vi "Random Data one Line.vi"() -> ()   [LabVIEW 2025]
uses:
  <vilib>/numeric/Random Number (Range) DBL.vi
  <vilib>/Analysis/4window.llb/Gaussian Window (DBL).vi
  <vilib>/Analysis/2dsp.llb/Complex FFT.vi
  <vilib>/Analysis/1siggen.llb/Ramp Pattern by Samples.vi
  <extravilib>/ChannelInstances/Tag-cdb/Instantiate.vi
  <extravilib>/ChannelInstances/Tag-cdb/EndpointRead.vi
  <extravilib>/ChannelInstances/Tag-cdb/Endpoint.vi
  <vilib>/Analysis/NI_AALPro.lvlib
  <vilib>/Analysis/NI_AALBase.lvlib
  <extravilib>/ChannelInstances/Tag-cdb.lvlib
  <vilib>/Analysis/2dsp.llb/Resample (constant to constant, complex single-channel).vi
panel:
  in  "Zoom Range":dbl=100.0 format="%#_13g"
  in  "Wait Time":dbl(slide)=71.49146578212554 scale=1.0..500.0
  in  "Zoom Point Index":i32=13
  in  "Individual Plots \nPer Vector":bool=TRUE
  out "Waveform Graph 2":dbl[][](graph)
  out "XY Graph":cluster{"XY Graph - Light":cdb[]}[](graph)
  out "XY Graph 2":cluster{"XY Graph - Light":cdb[]}[](graph)
  out "Spectrum":dbl[][](graph)
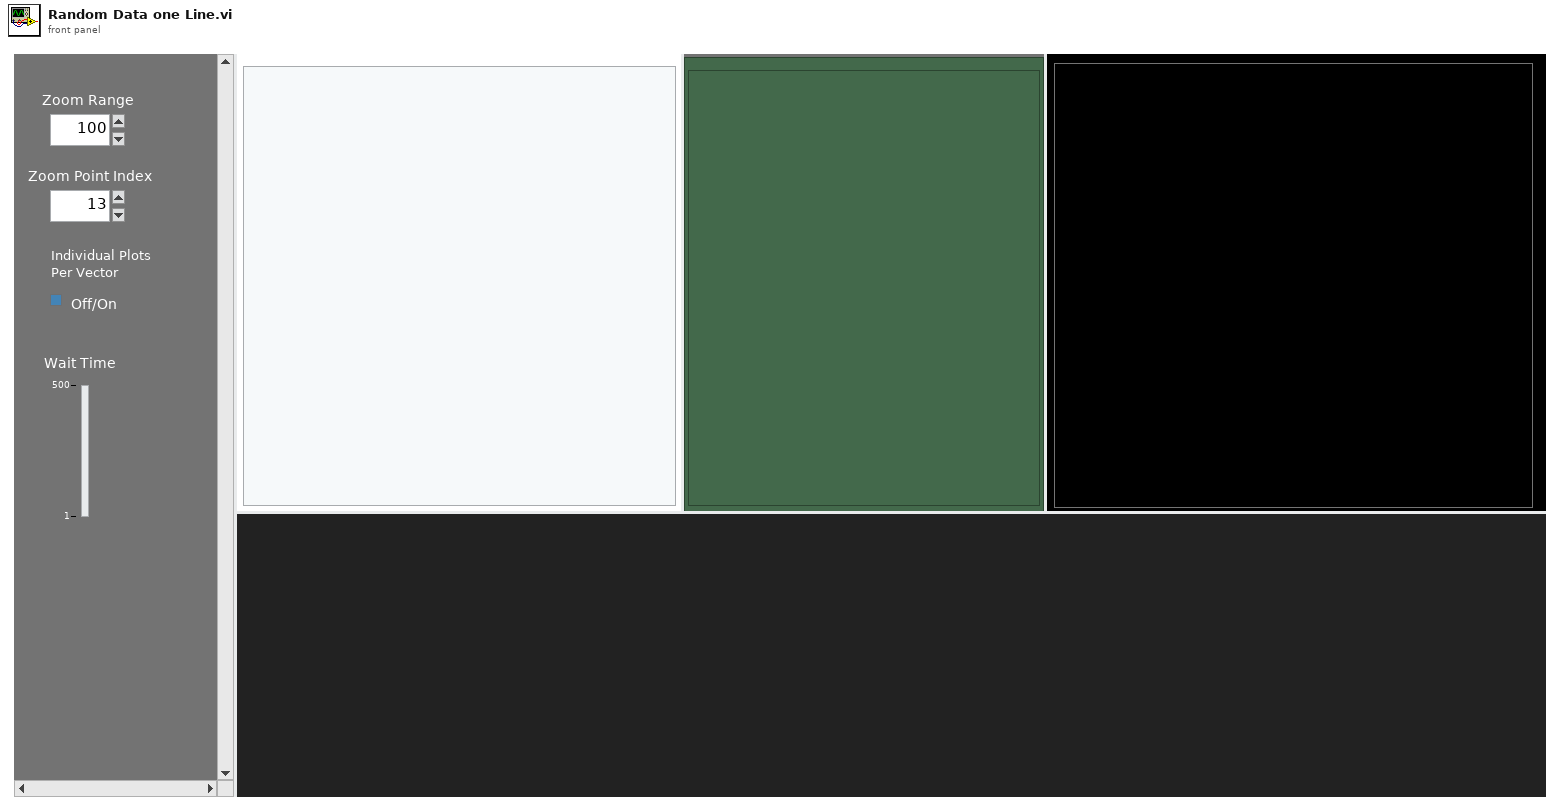
[diagram p1: front panel]
types:
  T1 = typedef "Tag-cdb.lvlib/))Channel.ctl" = refnum<queue>
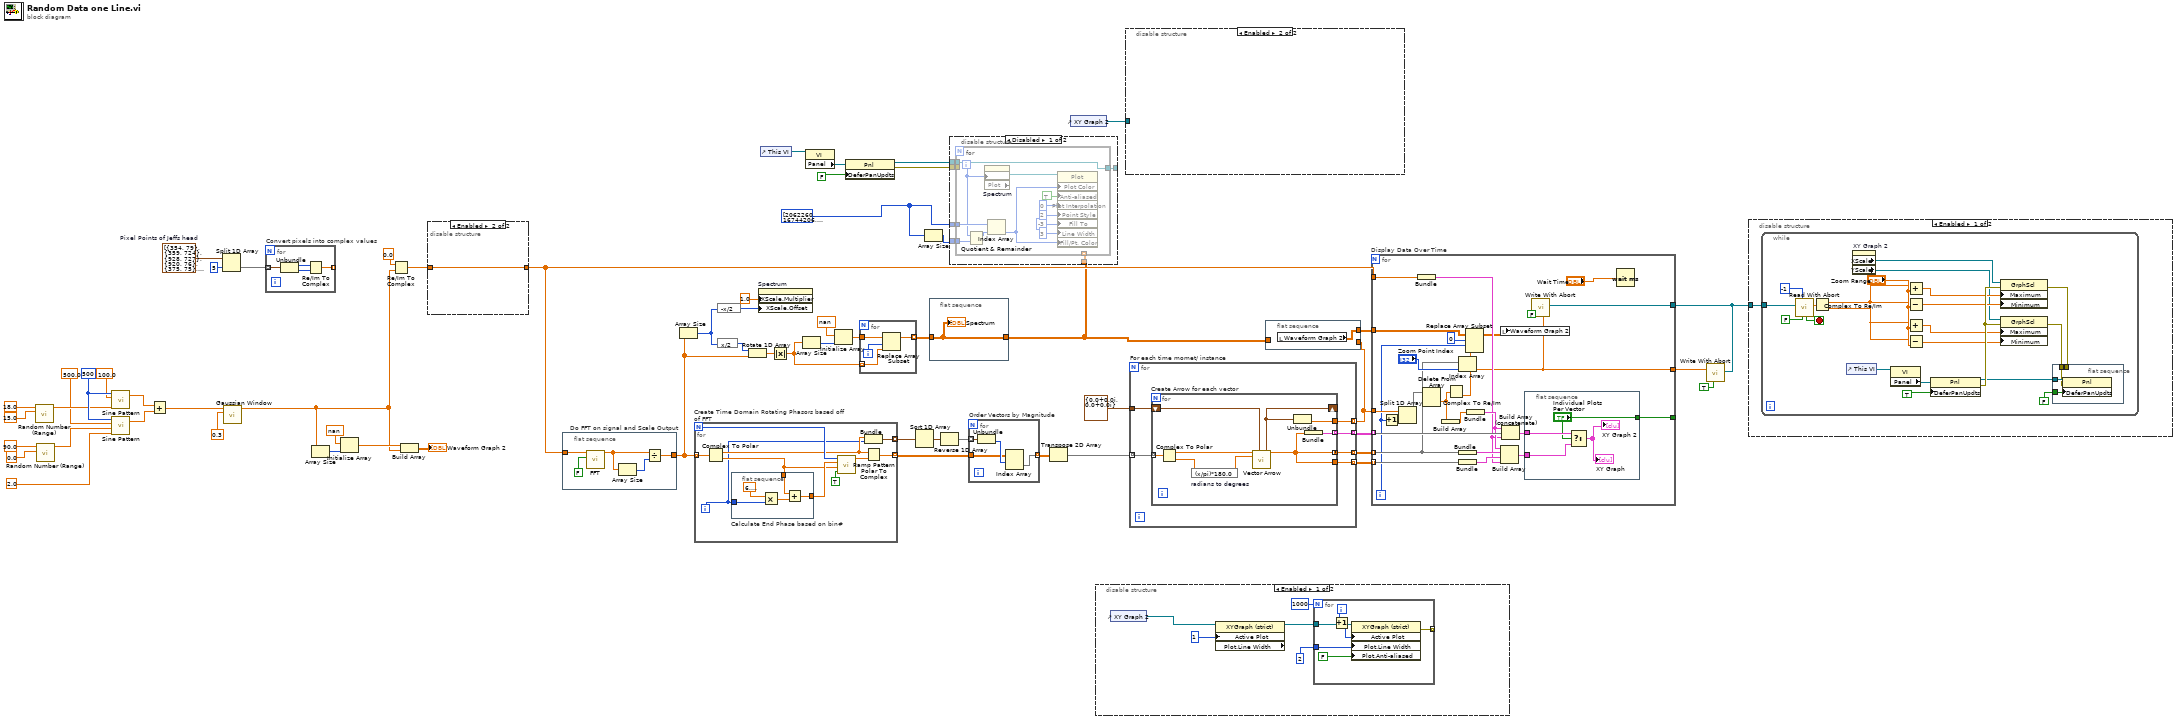
[diagram p0: block diagram]
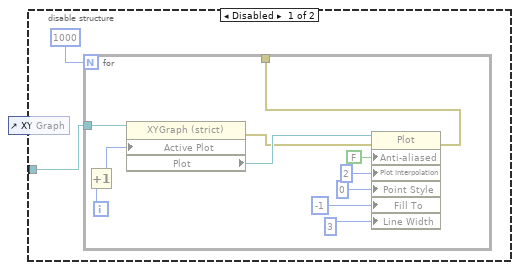
[diagram p3: hidden frame]
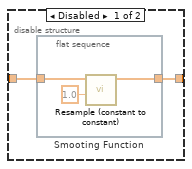
[diagram p5: hidden frame]
diagram:
  w2 = u32[] [2062260, 16744206, 2924588, 14034728, 9725885, 9197131, 14907330, 8355711, 12369186, 1556175] ("Array")
  w43 = 500 ("samples")
  w54 = cluster{"Horizontal":i32, "Vertical":i32}[] [{"Horizontal"=354, "Vertical"=79}, {"Horizontal"=359, "Vertical"=724}, {"Horizontal"=928, "Vertical"=727}, {"Horizontal"=920, "Vertical"=76}, {"Horizontal"=375, "Vertical"=75}, {"Horizontal"=348, "Vertical"=534}, {"Horizontal"=379, "Vertical"=519}, {"Horizontal"=407, "Vertical"=510}, {"Horizontal"=436, "Vertical"=501}, {"Horizontal"=463, "Vertical"=490}, {"Horizontal"=491, "Vertical"=484}, {"Horizontal"=514, "Vertical"=473}, {"Horizontal"=528, "Vertical"=466}, {"Horizontal"=536, "Vertical"=452}, {"Horizontal"=523, "Vertical"=437}, {"Horizontal"=518, "Vertical"=417}, {"Horizontal"=512, "Vertical"=396}, {"Horizontal"=508, "Vertical"=372}, {"Horizontal"=503, "Vertical"=348}, {"Horizontal"=490, "Vertical"=331}, {"Horizontal"=491, "Vertical"=315}, {"Horizontal"=502, "Vertical"=290}, {"Horizontal"=511, "Vertical"=302}, {"Horizontal"=520, "Vertical"=312}, {"Horizontal"=529, "Vertical"=324}, {"Horizontal"=531, "Vertical"=338}, {"Horizontal"=536, "Vertical"=353}, {"Horizontal"=547, "Vertical"=354}, {"Horizontal"=563, "Vertical"=359}, {"Horizontal"=570, "Vertical"=361}, {"Horizontal"=586, "Vertical"=363}, {"Horizontal"=595, "Vertical"=363}, {"Horizontal"=610, "Vertical"=363}, {"Horizontal"=617, "Vertical"=349}, {"Horizontal"=623, "Vertical"=335}, {"Horizontal"=629, "Vertical"=318}, {"Horizontal"=618, "Vertical"=309}, {"Horizontal"=601, "Vertical"=306}, {"Horizontal"=587, "Vertical"=303}, {"Horizontal"=567, "Vertical"=299}, {"Horizontal"=551, "Vertical"=301}, {"Horizontal"=539, "Vertical"=305}, {"Horizontal"=529, "Vertical"=306}, {"Horizontal"=520, "Vertical"=296}, {"Horizontal"=512, "Vertical"=281}, {"Horizontal"=506, "Vertical"=277}, {"Horizontal"=502, "Vertical"=269}, {"Horizontal"=508, "Vertical"=250}, {"Horizontal"=516, "Vertical"=232}, {"Horizontal"=525, "Vertical"=213}, {"Horizontal"=539, "Vertical"=188}, {"Horizontal"=547, "Vertical"=174}, {"Horizontal"=563, "Vertical"=162}, {"Horizontal"=579, "Vertical"=144}, {"Horizontal"=587, "Vertical"=136}, {"Horizontal"=610, "Vertical"=128}, {"Horizontal"=629, "Vertical"=129}, {"Horizontal"=656, "Vertical"=127}, {"Horizontal"=666, "Vertical"=131}, {"Horizontal"=697, "Vertical"=140}, {"Horizontal"=711, "Vertical"=143}, {"Horizontal"=745, "Vertical"=163}, {"Horizontal"=750, "Vertical"=169}, {"Horizontal"=757, "Vertical"=193}, {"Horizontal"=771, "Vertical"=200}, {"Horizontal"=767, "Vertical"=224}, {"Horizontal"=774, "Vertical"=238}, {"Horizontal"=779, "Vertical"=268}, {"Horizontal"=783, "Vertical"=284}, {"Horizontal"=765, "Vertical"=286}, {"Horizontal"=746, "Vertical"=291}, {"Horizontal"=737, "Vertical"=300}, {"Horizontal"=718, "Vertical"=302}, {"Horizontal"=696, "Vertical"=299}, {"Horizontal"=679, "Vertical"=302}, {"Horizontal"=655, "Vertical"=304}, {"Horizontal"=650, "Vertical"=306}, {"Horizontal"=636, "Vertical"=308}, {"Horizontal"=620, "Vertical"=309}, {"Horizontal"=643, "Vertical"=317}, {"Horizontal"=651, "Vertical"=334}, {"Horizontal"=656, "Vertical"=342}, {"Horizontal"=664, "Vertical"=358}, {"Horizontal"=674, "Vertical"=367}, {"Horizontal"=689, "Vertical"=360}, {"Horizontal"=712, "Vertical"=361}, {"Horizontal"=731, "Vertical"=353}, {"Horizontal"=738, "Vertical"=346}, {"Horizontal"=747, "Vertical"=326}, {"Horizontal"=744, "Vertical"=315}, {"Horizontal"=751, "Vertical"=304}, {"Horizontal"=759, "Vertical"=294}, {"Horizontal"=773, "Vertical"=291}, {"Horizontal"=785, "Vertical"=286}, {"Horizontal"=770, "Vertical"=296}, {"Horizontal"=778, "Vertical"=306}, {"Horizontal"=776, "Vertical"=317}, {"Horizontal"=775, "Vertical"=326}, {"Horizontal"=773, "Vertical"=340}, {"Horizontal"=771, "Vertical"=353}, {"Horizontal"=765, "Vertical"=360}, {"Horizontal"=762, "Vertical"=383}, {"Horizontal"=763, "Vertical"=406}, {"Horizontal"=761, "Vertical"=420}, {"Horizontal"=778, "Vertical"=434}, {"Horizontal"=782, "Vertical"=446}, {"Horizontal"=798, "Vertical"=459}, {"Horizontal"=811, "Vertical"=468}, {"Horizontal"=829, "Vertical"=476}, {"Horizontal"=847, "Vertical"=485}, {"Horizontal"=865, "Vertical"=489}, {"Horizontal"=878, "Vertical"=495}, {"Horizontal"=891, "Vertical"=500}, {"Horizontal"=903, "Vertical"=505}, {"Horizontal"=926, "Vertical"=511}, {"Horizontal"=912, "Vertical"=713}, {"Horizontal"=794, "Vertical"=706}, {"Horizontal"=812, "Vertical"=684}, {"Horizontal"=820, "Vertical"=665}, {"Horizontal"=829, "Vertical"=650}, {"Horizontal"=835, "Vertical"=631}, {"Horizontal"=844, "Vertical"=612}, {"Horizontal"=853, "Vertical"=594}, {"Horizontal"=859, "Vertical"=579}, {"Horizontal"=851, "Vertical"=571}, {"Horizontal"=840, "Vertical"=563}, {"Horizontal"=827, "Vertical"=556}, {"Horizontal"=837, "Vertical"=547}, {"Horizontal"=849, "Vertical"=536}, {"Horizontal"=851, "Vertical"=528}, {"Horizontal"=844, "Vertical"=519}, {"Horizontal"=840, "Vertical"=498}, {"Horizontal"=832, "Vertical"=485}, {"Horizontal"=829, "Vertical"=473}, {"Horizontal"=758, "Vertical"=419}, {"Horizontal"=760, "Vertical"=437}, {"Horizontal"=762, "Vertical"=465}, {"Horizontal"=755, "Vertical"=482}, {"Horizontal"=751, "Vertical"=506}, {"Horizontal"=744, "Vertical"=525}, {"Horizontal"=739, "Vertical"=547}, {"Horizontal"=731, "Vertical"=561}, {"Horizontal"=726, "Vertical"=580}, {"Horizontal"=723, "Vertical"=604}, {"Horizontal"=719, "Vertical"=620}, {"Horizontal"=715, "Vertical"=637}, {"Horizontal"=706, "Vertical"=665}, {"Horizontal"=705, "Vertical"=683}, {"Horizontal"=701, "Vertical"=700}, {"Horizontal"=698, "Vertical"=709}, {"Horizontal"=694, "Vertical"=718}, {"Horizontal"=689, "Vertical"=722}, {"Horizontal"=676, "Vertical"=712}, {"Horizontal"=674, "Vertical"=695}, {"Horizontal"=667, "Vertical"=682}, {"Horizontal"=671, "Vertical"=666}, {"Horizontal"=660, "Vertical"=646}, {"Horizontal"=664, "Vertical"=635}, {"Horizontal"=668, "Vertical"=624}, {"Horizontal"=675, "Vertical"=620}, {"Horizontal"=679, "Vertical"=623}, {"Horizontal"=692, "Vertical"=630}, {"Horizontal"=693, "Vertical"=633}, {"Horizontal"=698, "Vertical"=635}, {"Horizontal"=711, "Vertical"=628}, {"Horizontal"=721, "Vertical"=615}, {"Horizontal"=726, "Vertical"=586}, {"Horizontal"=746, "Vertical"=531}, {"Horizontal"=758, "Vertical"=482}, {"Horizontal"=753, "Vertical"=456}, {"Horizontal"=740, "Vertical"=475}, {"Horizontal"=727, "Vertical"=490}, {"Horizontal"=713, "Vertical"=503}, {"Horizontal"=696, "Vertical"=531}, {"Horizontal"=683, "Vertical"=529}, {"Horizontal"=671, "Vertical"=538}, {"Horizontal"=659, "Vertical"=550}, {"Horizontal"=642, "Vertical"=552}, {"Horizontal"=628, "Vertical"=553}, {"Horizontal"=602, "Vertical"=550}, {"Horizontal"=592, "Vertical"=529}, {"Horizontal"=586, "Vertical"=528}, {"Horizontal"=579, "Vertical"=519}, {"Horizontal"=570, "Vertical"=508}, {"Horizontal"=564, "Vertical"=492}, {"Horizontal"=557, "Vertical"=481}, {"Horizontal"=553, "Vertical"=470}, {"Horizontal"=548, "Vertical"=456}, {"Horizontal"=540, "Vertical"=468}, {"Horizontal"=541, "Vertical"=485}, {"Horizontal"=542, "Vertical"=508}, {"Horizontal"=539, "Vertical"=527}, {"Horizontal"=544, "Vertical"=555}, {"Horizontal"=543, "Vertical"=588}, {"Horizontal"=539, "Vertical"=614}, {"Horizontal"=539, "Vertical"=631}, {"Horizontal"=539, "Vertical"=656}, {"Horizontal"=542, "Vertical"=673}, {"Horizontal"=539, "Vertical"=687}, {"Horizontal"=545, "Vertical"=712}, {"Horizontal"=542, "Vertical"=723}, {"Horizontal"=547, "Vertical"=727}, {"Horizontal"=572, "Vertical"=724}, {"Horizontal"=578, "Vertical"=696}, {"Horizontal"=578, "Vertical"=682}, {"Horizontal"=586, "Vertical"=659}, {"Horizontal"=588, "Vertical"=638}, {"Horizontal"=593, "Vertical"=613}, {"Horizontal"=601, "Vertical"=601}, {"Horizontal"=609, "Vertical"=614}, {"Horizontal"=613, "Vertical"=626}, {"Horizontal"=625, "Vertical"=640}, {"Horizontal"=614, "Vertical"=670}, {"Horizontal"=610, "Vertical"=680}, {"Horizontal"=604, "Vertical"=701}, {"Horizontal"=604, "Vertical"=706}, {"Horizontal"=602, "Vertical"=710}, {"Horizontal"=597, "Vertical"=718}, {"Horizontal"=596, "Vertical"=718}, {"Horizontal"=597, "Vertical"=718}, {"Horizontal"=596, "Vertical"=717}, {"Horizontal"=596, "Vertical"=717}, {"Horizontal"=597, "Vertical"=715}, {"Horizontal"=598, "Vertical"=709}, {"Horizontal"=598, "Vertical"=709}, {"Horizontal"=597, "Vertical"=709}, {"Horizontal"=573, "Vertical"=709}, {"Horizontal"=585, "Vertical"=684}, {"Horizontal"=591, "Vertical"=655}, {"Horizontal"=597, "Vertical"=623}, {"Horizontal"=599, "Vertical"=596}, {"Horizontal"=588, "Vertical"=609}, {"Horizontal"=577, "Vertical"=631}, {"Horizontal"=566, "Vertical"=639}, {"Horizontal"=539, "Vertical"=591}, {"Horizontal"=545, "Vertical"=484}, {"Horizontal"=563, "Vertical"=510}, {"Horizontal"=582, "Vertical"=478}, {"Horizontal"=595, "Vertical"=486}, {"Horizontal"=606, "Vertical"=492}, {"Horizontal"=641, "Vertical"=500}, {"Horizontal"=652, "Vertical"=495}, {"Horizontal"=660, "Vertical"=496}, {"Horizontal"=684, "Vertical"=488}, {"Horizontal"=695, "Vertical"=478}, {"Horizontal"=701, "Vertical"=471}, {"Horizontal"=695, "Vertical"=427}, {"Horizontal"=683, "Vertical"=432}, {"Horizontal"=660, "Vertical"=437}, {"Horizontal"=651, "Vertical"=441}, {"Horizontal"=635, "Vertical"=438}, {"Horizontal"=615, "Vertical"=436}, {"Horizontal"=605, "Vertical"=434}, {"Horizontal"=594, "Vertical"=429}, {"Horizontal"=587, "Vertical"=422}, {"Horizontal"=591, "Vertical"=415}, {"Horizontal"=603, "Vertical"=422}, {"Horizontal"=619, "Vertical"=424}, {"Horizontal"=629, "Vertical"=424}, {"Horizontal"=645, "Vertical"=423}, {"Horizontal"=653, "Vertical"=422}, {"Horizontal"=661, "Vertical"=422}, {"Horizontal"=679, "Vertical"=421}, {"Horizontal"=686, "Vertical"=419}, {"Horizontal"=687, "Vertical"=418}, {"Horizontal"=705, "Vertical"=409}, {"Horizontal"=696, "Vertical"=390}, {"Horizontal"=687, "Vertical"=382}, {"Horizontal"=676, "Vertical"=378}, {"Horizontal"=664, "Vertical"=386}, {"Horizontal"=648, "Vertical"=397}, {"Horizontal"=642, "Vertical"=397}, {"Horizontal"=626, "Vertical"=394}, {"Horizontal"=616, "Vertical"=389}, {"Horizontal"=605, "Vertical"=383}, {"Horizontal"=606, "Vertical"=375}, {"Horizontal"=616, "Vertical"=361}, {"Horizontal"=624, "Vertical"=344}, {"Horizontal"=631, "Vertical"=329}, {"Horizontal"=641, "Vertical"=322}, {"Horizontal"=648, "Vertical"=330}, {"Horizontal"=657, "Vertical"=349}, {"Horizontal"=669, "Vertical"=360}, {"Horizontal"=681, "Vertical"=369}]  # Pixel Points of Jeffs head
  n1 = call-poly <vilib>:"Random Number (Range).vi"("lower bound (0)"=15.0, "upper bound (100)"=18.0) -> ("number"=w38:dbl)  [unwired: 9 in]
  n2 = call-poly <vilib>:"Random Number (Range).vi"("lower bound (0)"=0.0, "upper bound (100)"=90.0) -> ("number"=w22:dbl)  [unwired: 9 in]
  n3 = call <vilib>:"Sine Pattern.vi"("cycles"=w38, "amplitude"=100.0, "samples"=w43) -> ("Sinusoidal Pattern"=w41:dbl[])  [unwired: 1 in, 1 out]
  n4 = call <vilib>:"Sine Pattern.vi"("cycles"=2.0, "phase(degrees)"=w22, "amplitude"=500.0, "samples"=w43) -> ("Sinusoidal Pattern"=w40:dbl[])  [unwired: 1 out]
  n5 = Add(x=w41, y=w40) -> (x+y=w26:dbl[])
  n6 = Split 1D Array(array=w54, index=5) -> (second subarray=w53:cluster{"Horizontal":i32, "Vertical":i32}[])  [unwired: 1 out]
  n7 = call-poly <vilib>:"Gaussian Window.vi"("standard deviation"=0.3, "X"=w26) -> ("Windowed X"=w17:dbl[])  [unwired: 8 in, 1 out]
  n8 = for "Convert pixels into complex values" {
    tunnel: w53 -> [w64] mode=indexing
    tunnel: [w61] -> _ mode=indexing
    n9 = Unbundle(w64) -> ("Horizontal"=w63:i32, "Vertical"=w62:i32)
    n10 = Re/Im To Complex(1:w62, 2:w63) -> (0:w61:cdb)
  }
  n11 = Array Size(array=w17) -> (size(s)=w18:i32)
  n12 = Initialize Array(nan ("element"), w18) -> (w19:dbl[])
  n13 = Re/Im To Complex(1:w17, 2:0.0 ("cycles")) -> (0:w16:cdb[])
  n14 = Build Array(w19, w17) -> (→"Waveform Graph 2":dbl[][])
  n15 = disable-structure shown="Enabled" {
    disable-tunnel: w16 -> [w66 w70]
    disable-tunnel: [w65 w70] -> w55
    frame Disabled {
      n16 = flat-sequence "Smooting Function" {
        tunnel: w66 -> [w69]
        tunnel: [w67] -> w65
        frame #0 {
          n17 = call-poly <vilib>:"Resample (constant to constant).vi"("dt"=1.0, "X"=w69) -> ("Y"=w67:cdb[])  [unwired: 7 in, 2 out]
        }
      }
    }
    frame Enabled {
    }
  }
  n18 = flat-sequence "Do FFT on signal and Scale Output" {
    tunnel: [w74] -> w35
    tunnel: w55 -> [w73]
    frame #0 {
      n19 = call-poly <vilib>:"FFT.vi"("shift?"=FALSE, "X"=w73) -> ("FFT {X}"=w75:cdb[])  [unwired: 8 in, 1 out]
      n20 = Array Size(array=w75) -> (size(s)=w72:i32)
      n21 = Divide(x=w75, y=w72) -> (x/y=w74:cdb[])
    }
  }
  n22 = Array Size(array=w35) -> (size(s)=w10:i32)
  n23 = for "Create Time Domain Rotating Phasors based off of FFT" {
    N -> [w83]
    tunnel: w35 -> [w85] mode=indexing
    tunnel: [w81] -> w49 mode=indexing
    tunnel: [w76] -> w51 mode=indexing
    i -> [w77]
    n24 = Complex To Polar(r * e^(i*theta)=w85) -> (r=w78:dbl, theta=w79:dbl)
    n25 = flat-sequence "Calculate End Phase based on bin#" {
      tunnel: [w88] -> w84
      tunnel: w77 -> [w87]
      tunnel: w79 -> [w86]
      frame #0 {
        n26 = Multiply(x=6.283185307179586, y=w87) -> (x*y=w89:dbl)
        n27 = Add(x=w86, y=w89) -> (x+y=w88:dbl)
      }
    }
    n28 = call-poly <vilib>:"Ramp Pattern.vi"("exclude end?"=TRUE, "start"=w79, "end"=w84, "samples"=w83) -> ("Ramp Pattern"=w82:dbl[])  [unwired: 6 in, 1 out]
    n29 = Bundle(w78, w77) -> (w76:cluster{dbl, i32})  [unwired: 1 in]
    n30 = Polar To Complex(1:w82, 2:w78) -> (0:w81:cdb[])
  }
  n31 = expression code="-x/2"(w10) -> (w33:i32)
  n32 = expression code="x/2"(w10) -> (w12:i32)
  n33 = Rotate 1D Array(1:w35, 2:w12) -> (0:w34:cdb[])
  n34 = property on="Spectrum" class="WFGraph (strict)"("XScale.Multiplier"=1.0 ("X Scale.Offset and Multiplier:Multiplier"), "XScale.Offset"=w33) -> ()  [unwired: 2 in, 2 out]
  n35 = control-ref of="This VI"() -> (w6:refnum<vi>)
  n36 = Absolute Value(x=w34) -> (abs(x)=w11:dbl[])
  n37 = Array Size(array=w11) -> (size(s)=w30:i32)
  n38 = property class="VI"(reference=w6) -> ("Panel"=w8:refnum<vi>)  [unwired: 1 in, 2 out]
  n39 = Initialize Array(nan ("element"), w30) -> (w28:dbl[])
  n40 = property class="Pnl"(reference=w8, "DeferPanUpdts"=FALSE ("Defer Panel Updates")) -> (reference out=w4:refnum<vi>, error out=w5:errorcluster)  [unwired: 1 in]
  n41 = for {
    tunnel: w11 -> [w93] mode=indexing
    tunnel: [w91] -> w32 mode=indexing
    tunnel: w28 -> [w94]
    i -> [w92]
    n42 = Replace Array Subset(array=w94, new element=w93, index=w92) -> (w91:dbl[])
  }
  n43 = Sort 1D Array(array=w51) -> (sorted array=w50:cluster{dbl, i32}[])
  n44 = Array Size(array=w2) -> (size(s)=w9:i32)
  n45 = flat-sequence {
    tunnel: w32 -> [w95]
    tunnel: [w95] -> w3
    frame #0 {
      "Spectrum" <- w95
    }
  }
  n46 = Reverse 1D Array(array=w50) -> (reversed array=w47:cluster{dbl, i32}[])
  n47 = disable-structure shown="Disabled" {
    disable-tunnel: w3 -> [w101 _]
    disable-tunnel: w2 -> [w100 _]
    disable-tunnel: w9 -> [w99 _]
    disable-tunnel: w5 -> [w98 _]
    disable-tunnel: [w97 _] -> _
    disable-tunnel: w4 -> [w96 _]
    frame Disabled {
      n48 = for {
        tunnel: w101 -> [_] mode=indexing
        tunnel: w100 -> [w108]
        tunnel: w99 -> [w107]
        tunnel: w98 -> [_]
        tunnel: [w105] -> w97
        tunnel: w96 -> [w105]
        i -> [w104]
        n49 = Quotient & Remainder(x=w104, y=w107) -> (x-y*floor(x/y)=w106:i32)  [unwired: 1 out]
        n50 = property on="Spectrum" class="WFGraph (strict)"("Active Plot"=w104) -> ("Plot"=w113:refnum<vi>)  [unwired: 2 in, 2 out]
        n51 = Index Array(array=w108, index=w106) -> (element=w102:u32)
        n52 = property class="Plot"(reference=w113, "Plot Color"=w102, "Anti-aliased"=TRUE, "Plot Interpolation"=u8 0, "Point Style"=u8 2, "Fill To"=i16 -3, "Line Width"=u8 3, "Fill/Pt. Color"=w102) -> ()  [unwired: 1 in, 2 out]
      }
    }
    frame Enabled {
    }
  }
  n53 = for "Order Vectors by Magnitude" {
    tunnel: w47 -> [w117] mode=indexing
    tunnel: w49 -> [w115]
    tunnel: [w114] -> w48 mode=indexing
    n54 = Unbundle(w117) -> (w116:i32)  [unwired: 1 out]
    n55 = Index Array(array=w115, index (row)=w116) -> (element=w114:cdb[])  [unwired: 1 in]
  }
  n56 = Transpose 2D Array(2D array=w48) -> (transposed array=w59:cdb[][])
  n57 = control-ref of="XY Graph 2"() -> (w1:refnum<vi>)
  n58 = disable-structure shown="Enabled" {
    frame Enabled {
      n59 = control-ref of="XY Graph 2"() -> (w119:refnum<vi>)
      n60 = property class="XYGraph (strict)" props=["Active Plot", "Plot", "Line Width"](reference=w119, "Active Plot"=u32 1) -> (reference out=w121:refnum<vi>)  [unwired: 1 in, 2 out]
      n61 = for {
        N: 1000 -> [_]
        tunnel: w121 -> [w128]
        tunnel: [w127] -> _ mode=indexing
        tunnel: u8 2 ("Plot.Line Width") -> [w125]
        i -> [w126]
        n62 = Increment(x=w126) -> (x+1=w123:i32)
        n63 = property class="XYGraph (strict)"(reference=w128, "Active Plot"=w123, "Plot.Line Width"=w125, "Plot.Anti-aliased"=FALSE) -> (error out=w127:errorcluster)  [unwired: 1 in, 1 out]
      }
    }
    frame Disabled {
    }
  }
  n64 = disable-structure shown="Enabled" {
    disable-tunnel: w1 -> [w129 _]
    frame Disabled {
      n65 = control-ref of="XY Graph"() -> ()  [unwired: 1 out]
      n66 = for {
        N: 1000 -> [_]
        tunnel: w129 -> [w141]
        tunnel: [w132] -> _
        i -> [w140]
        n67 = Increment(x=w140) -> (x+1=w131:i32)
        n68 = property on="Property Node" class="XYGraph (strict)"(reference=w141, "Active Plot"=w131) -> (error out=w133:errorcluster, "Plot"=w134:refnum<vi>)  [unwired: 1 in, 1 out]
        n69 = property class="Plot"(reference=w134, error in=w133, "Anti-aliased"=FALSE, "Plot Interpolation"=u8 2, "Point Style"=u8 0, "Fill To"=i16 -1, "Line Width"=u8 3) -> (error out=w132:errorcluster)  [unwired: 1 out]
      }
    }
    frame Enabled {
    }
  }
  n70 = for "For each time momet/ instance" {
    tunnel: cluster{"Initial":cdb, "Endpoint":cdb} {"Initial"=0.0+0.0i, "Endpoint"=0.0+0.0i} ("Resultant Vector") -> [w147]
    tunnel: w59 -> [w145] mode=indexing
    tunnel: [w146] -> w58 mode=indexing
    tunnel: [w144] -> w57 mode=indexing
    tunnel: [w143] -> w56 mode=indexing
    tunnel: [w142] -> w24 mode=indexing
    n71 = for "Create Arrow for each vector" {
      tunnel: [w156] -> w146 mode=indexing
      shift-right: [w149] -> _
      shift-left: w147 -> [w155]
      tunnel: w145 -> [w154] mode=indexing
      tunnel: [w153] -> w144 mode=concatenating
      tunnel: [w153] -> w143
      tunnel: [w148] -> w142
      n72 = Complex To Polar(r * e^(i*theta)=w154) -> (r=w152:dbl, theta=w151:dbl)
      n73 = expression code="(x/pi)*180.0" "radians to degrees"(w151) -> (w150:dbl)
      n74 = call "Vector Arrow.vi"("Magnitude"=w152, "Initial Vector"=w155, "Phase, deg"=w150) -> ("Resultant Vector"=w149:cluster{"Initial":cdb, "Endpoint":cdb}, "XY Graph - Light"=w153:cdb[])  [unwired: 11 in]
      n75 = Unbundle(w149) -> ("Endpoint"=w148:cdb)  [unwired: 1 out]
      n76 = Bundle("XY Graph - Light"=w153) -> (w156:cluster{"XY Graph - Light":cdb[]})  [unwired: 1 in]
    }
  }
  n77 = flat-sequence {
    tunnel: [w157] -> w25
    tunnel: w24 -> [_]
    tunnel: w3 -> [_]
    frame #0 {
      n78 = local read "Waveform Graph 2"() -> (w157:dbl[][])
    }
  }
  n79 = for "Display Data Over Time" {
    tunnel: w58 -> [w180] mode=indexing
    tunnel: w57 -> [w168] mode=indexing
    tunnel: w55 -> [w182]
    tunnel: w56 -> [w169] mode=indexing
    tunnel: w24 -> [w177]
    tunnel: [w173] -> w44
    tunnel: [w172] -> w46
    tunnel: w25 -> [w160]
    tunnel: [w158] -> _
    i -> [w164]
    n80 = Increment(x=w164) -> (x+1=w176:i32)
    n81 = Split 1D Array(array=w177, index=w176) -> (first subarray=w167:cdb[])  [unwired: 1 out]
    n82 = Bundle(w182) -> (w174:cluster{cdb[]})  [unwired: 1 in]
    n83 = Delete From Array(array=w167) -> (deleted portion=w163:cdb)  [unwired: 2 in, 1 out]
    n84 = Build Array(w163) -> (w166:cdb[])
    n85 = Complex To Re/Im(x + iy=w163) -> (y=w162:dbl)  [unwired: 1 out]
    n86 = Bundle("XY Graph - Light"=w168) -> (w183:cluster{"XY Graph - Light":cdb[]})  [unwired: 1 in]
    n87 = Bundle("XY Graph - Light"=w169) -> (w181:cluster{"XY Graph - Light":cdb[]})  [unwired: 1 in]
    n88 = Index Array(array=w168, index="Zoom Point Index") -> (element=w172:cdb)
    n89 = Replace Array Subset(array=w160, new element=w162, index (row)=0, index (col)=w164) -> (w161:dbl[][])
    n90 = Bundle(w166) -> (w175:cluster{cdb[]})  [unwired: 1 in]
    n91 = local write "Waveform Graph 2"(w161) -> ()
    n92 = Build Array(w175, w183, w181, w174) -> (w178:cluster{"XY Graph - Light":cdb[]}[])
    n93 = Build Array (concatenate)(w175, w180, w174) -> (w179:cluster{"XY Graph - Light":cdb[]}[])
    n94 = flat-sequence {
      tunnel: w179 -> [w187]
      tunnel: w178 -> [w186]
      tunnel: ["Individual Plots \nPer Vector"] -> w158
      frame #0 {
        n95 = Select(t=w187, s="Individual Plots \nPer Vector", f=w186) -> (s? t:f=→"XY Graph" →"XY Graph 2":cluster{"XY Graph - Light":cdb[]}[])
      }
    }
    n96 = call <extravilib>:"Write With Abort.vi"("abort"=FALSE, "element"=w172) -> ("channel"=w173:T1)  [unwired: 7 in, 2 out]
    n97 = Wait (ms)(milliseconds to wait="Wait Time") -> ()  [unwired: 1 out]
  }
  n98 = call <extravilib>:"Write With Abort.vi"("channel"=w44, "abort"=TRUE, "element"=w46) -> ()  [unwired: 7 in, 2 out]
  n99 = disable-structure shown="Enabled" {
    disable-tunnel: w44 -> [w188 _]
    frame Enabled {
      n100 = while {
        tunnel: w188 -> [w202]
        stop <- w201 stop-if-true
        n101 = call <extravilib>:"Read With Abort.vi"("abort"=FALSE, "timeout in ms (0)"=-1, "channel"=w202) -> ("element"=w190:cdb, "aborted?"=w201:bool)  [unwired: 6 in, 1 out]
        n102 = Complex To Re/Im(x + iy=w190) -> (x=w200:dbl, y=w199:dbl)
        n103 = control-ref of="This VI"() -> (w191:refnum<vi>)
        n104 = property on="XY Graph 2" class="XYGraph (strict)"() -> ("XScale"=w204:refnum<vi>, "YScale"=w205:refnum<vi>)  [unwired: 2 in, 2 out]
        n105 = property class="VI"(reference=w191) -> ("Panel"=w198:refnum<vi>)  [unwired: 1 in, 2 out]
        n106 = Add(x=w200, y="Zoom Range") -> (x+y=w209:dbl)
        n107 = Subtract(x=w200, y="Zoom Range") -> (x-y=w208:dbl)
        n108 = Add(x=w199, y="Zoom Range") -> (x+y=w207:dbl)
        n109 = Subtract(x=w199, y="Zoom Range") -> (x-y=w206:dbl)
        n110 = property class="Pnl"(reference=w198, "DeferPanUpdts"=TRUE ("Defer Panel Updates")) -> (reference out=w196:refnum<vi>, error out=w210:errorcluster)  [unwired: 1 in]
        n111 = property class="GrphScl"(reference=w204, error in=w210, "Maximum"=w209, "Minimum"=w208) -> (error out=w194:errorcluster)  [unwired: 1 out]
        n112 = property class="GrphScl"(reference=w205, error in=w210, "Maximum"=w207, "Minimum"=w206) -> (error out=w195:errorcluster)  [unwired: 1 out]
        n113 = flat-sequence {
          tunnel: w196 -> [w213]
          tunnel: w195 -> [w212]
          tunnel: w194 -> [_]
          tunnel: FALSE ("DeferPanUpdts") -> [w211]
          frame #0 {
            n114 = property class="Pnl"(reference=w213, error in=w212, "DeferPanUpdts"=w211) -> ()  [unwired: 2 out]
          }
        }
      }
    }
    frame Disabled {
    }
  }
